vi "Test Schema Selector Update.vi"(8 "error in (no error)":errorcluster, 9 "Schema":string, 10 "Test Log":refnum<vi>, 11 "Post Analysis in":refnum<class "Post Analysis.lvclass">) -> (0 "error out":errorcluster, 3 "Post Analysis out":refnum<class "Post Analysis.lvclass">)   [LabVIEW 2023, in "Data Analysis.lvlib" / "Post Analysis.lvlib" / "Post Analysis.lvclass"]
uses:
  Post Analysis.lvclass
  Post Analysis.lvclass/Post Analysis.ctl
  Test Info/Test Info Messages/Test Log Schema Update Msg/Test Log Schema Update Msg.lvclass/Test Log Schema Update Msg.ctl
  <vilib>/ActorFramework/Message Enqueuer/Message Enqueuer.lvclass/Message Enqueuer.ctl
  FE FF Frame/FE FF Frame Messages/Schema Update Msg/Schema Update Msg.lvclass/Schema Update Msg.ctl
  Import Export/Import Export Messages/Show Tables Msg/Show Tables Msg.lvclass/Show Tables Msg.ctl
  <vilib>/ActorFramework/Message Enqueuer/Enqueue.vi
  Test Info/Test Info Messages/Test Log Schema Update Msg/Test Log Schema Update Msg.lvclass
  C:/Program Files/National Instruments/LabVIEW 2023/vi.lib/ActorFramework/Message/Message.lvclass
  Error Log/Error Log Messages/Initialise the Error log Based on Cycle number Msg/Initialise the Error log Based on Cycle number Msg.lvclass
  FE FF Frame/FE FF Frame Messages/Schema Update Msg/Schema Update Msg.lvclass
  Signal Analysis/Signal Analysis Messages/Signal Name Update Msg/Signal Name Update Msg.lvclass
  Import Export/Import Export Messages/Show Tables Msg/Show Tables Msg.lvclass
  <vilib>/ActorFramework/Message Priority Queue/Priority Enqueue.vi
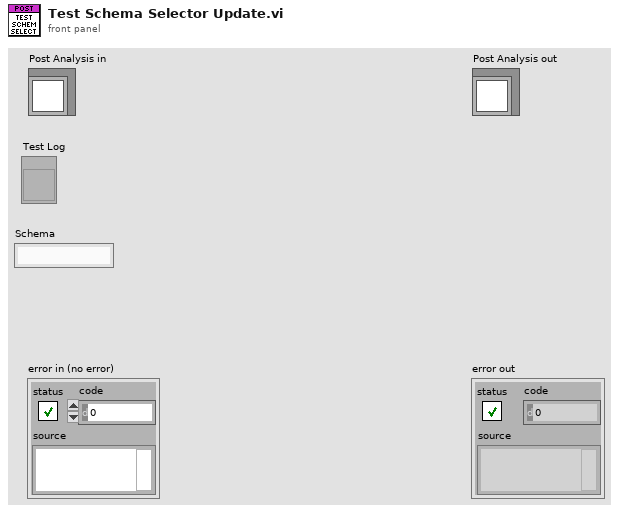
[diagram p1: front panel]
types:
  T1 = enum8{"Enabled", "Disabled", "Disabled and Grayed Out"}
  T2 = enum32{"Test Info", "Error Log", "FE/FF Frame", "Signal Analysis", "Export", "Database", "Info"}
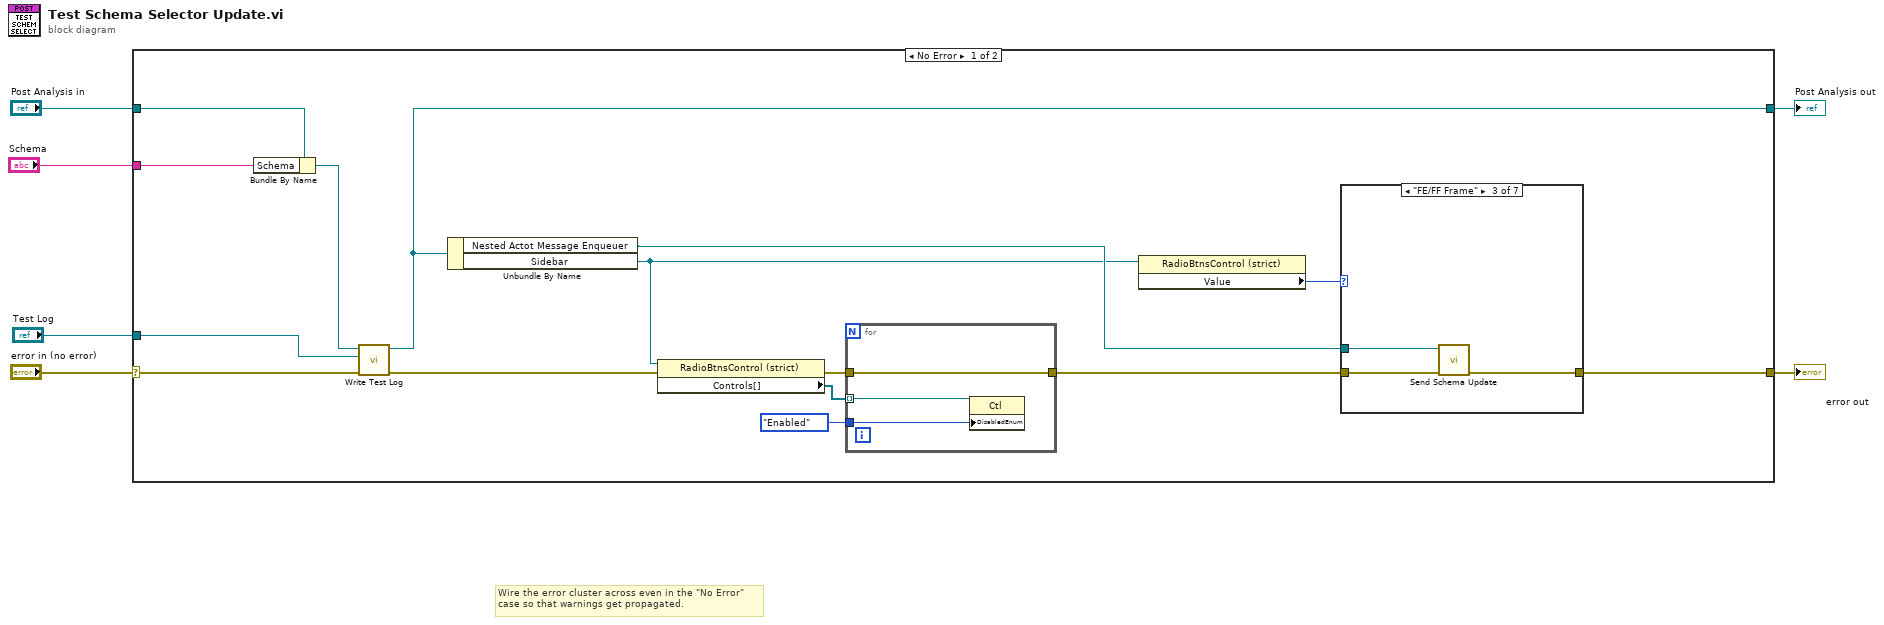
[diagram p0: block diagram]
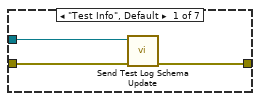
[diagram p2: hidden frame]
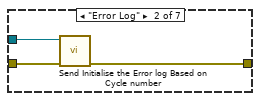
[diagram p3: hidden frame]
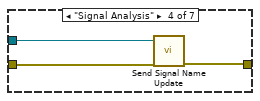
[diagram p4: hidden frame]
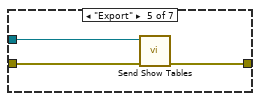
[diagram p5: hidden frame]
diagram:
  # "Wire the error cluster across even in the \"No Error\"\ncase so that warnings get propagated."
  n1 = case shown="No Error" "error in (no error)" {
    selector: "error in (no error)" -> [w20 w43]
    tunnel: [w17 w43] -> w5
    tunnel: [w19 w42] -> w3
    tunnel: "Post Analysis in" -> [w16 w42]
    tunnel: "Test Log" -> [w21 _]
    tunnel: "Schema" -> [w7 _]
    frame No Error {
      n2 = Bundle By Name(cluster=w16, "Schema"=w7) -> (w15:refnum<class "Post Analysis.lvclass">)
      n3 = call "Write Test Log.vi"("error in (no error)"=w20, "Test Log"=w21, "Post Analysis in"=w15) -> ("error out"=w14:errorcluster, "Post Analysis out"=w19:refnum<class "Post Analysis.lvclass">)  [unwired: 7 in]
      n4 = Unbundle By Name(w19) -> ("Nested Actot Message Enqueuer"=w13:refnum<class "Message Enqueuer.lvclass">, "Sidebar"=w12:refnum<vi>)
      n5 = property class="RadioBtnsControl (strict)"(reference=w12, error in=w14) -> (error out=w9:errorcluster, "Controls[]"=w11:refnum<vi>[])  [unwired: 1 out]
      n6 = for {
        tunnel: w11 -> [w24] mode=indexing
        tunnel: T1."Enabled" ("Disabled") -> [w23]
        tunnel: w9 -> [w22]
        tunnel: [w22] -> w8
        n7 = property class="Ctl"(reference=w24, "DisabledEnum"=w23) -> ()  [unwired: 1 in, 2 out]
      }
      n8 = property class="RadioBtnsControl (strict)"(reference=w12) -> ("Value"=w18:T2)  [unwired: 1 in, 2 out]
      n9 = case shown="\"FE/FF Frame\"" w18 {
        tunnel: w8 -> [w26 w29 w33 w35 w39 w40 w41]
        tunnel: [w25 w28 w32 w34 w38 w40 w41] -> w17
        tunnel: w13 -> [w27 w30 w31 w36 w37 _ _]
        frame "Test Info", Default {
          n10 = call "Send Test Log Schema Update.vi"("error in (no error)"=w26, "Message Enqueuer"=w27) -> ("error out"=w25:errorcluster)  [unwired: 8 in, 1 out]
        }
        frame "Error Log" {
          n11 = call "Send Initialise the Error log Based on Cycle number.vi"("error in (no error)"=w29, "Message Enqueuer"=w30) -> ("error out"=w28:errorcluster)  [unwired: 8 in, 1 out]
        }
        frame "FE/FF Frame" {
          n12 = call "Send Schema Update.vi"("error in (no error)"=w33, "Message Enqueuer"=w31) -> ("error out"=w32:errorcluster)  [unwired: 8 in, 1 out]
        }
        frame "Signal Analysis" {
          n13 = call "Send Signal Name Update.vi"("error in (no error)"=w35, "Message Enqueuer"=w36) -> ("error out"=w34:errorcluster)  [unwired: 8 in, 1 out]
        }
        frame "Export" {
          n14 = call "Send Show Tables.vi"("error in (no error)"=w39, "Message Enqueuer"=w37) -> ("error out"=w38:errorcluster)  [unwired: 8 in, 1 out]
        }
        frame "Info" {
        }
        frame "Database" {
        }
      }
    }
    frame Error {
    }
  }
  "error out" <- w5
  "Post Analysis out" <- w3
